vi "App - analyze RUS V6.vi"() -> ()   [LabVIEW 2021] (continued)
"temperature str"="160.67400", "file path"=path "D:/Data/Ultrasound/LSCO/LSCO22__130814c/5_Cooling_2nd_try/September_2014/091614/160.67400K_500_2500_2.10000V_0.00000T_Sep16-2014__16-59-49_001_091614.bin", "last mod"=timestamp(3493745989 s since 1904-01-01), "file name str"="D:\\Data\\Ultrasound\\LSCO\\LSCO22__130814c\\5_Cooling_2nd_try\\September_2014\\091614\\160.67400K_500_2500_2.10000V_0.00000T_Sep16-2014__16-59-49_001_091614.bin", "mod time(min)"=58229099.81666667, "file format"=enum."binary", "power(V)"=2.1, "Magn Field(T) "=0.0}, {"temperature"=160.342, "temperature str"="160.34200", "file path"=path "D:/Data/Ultrasound/LSCO/LSCO22__130814c/5_Cooling_2nd_try/September_2014/091614/160.34200K_500_2500_2.10000V_0.00000T_Sep16-2014__17-01-09_001_091614.bin", "last mod"=timestamp(3493746069 s since 1904-01-01), "file name str"="D:\\Data\\Ultrasound\\LSCO\\LSCO22__130814c\\5_Cooling_2nd_try\\September_2014\\091614\\160.34200K_500_2500_2.10000V_0.00000T_Sep16-2014__17-01-09_001_091614.bin", "mod time(min)"=58229101.15, "file format"=enum."binary", "power(V)"=2.1, "Magn Field(T) "=0.0}, {"temperature"=159.993, "temperature str"="159.99300", "file path"=path "D:/Data/Ultrasound/LSCO/LSCO22__130814c/5_Cooling_2nd_try/September_2014/091614/159.99300K_500_2500_2.10000V_0.00000T_Sep16-2014__17-02-28_001_091614.bin", "last mod"=timestamp(3493746148 s since 1904-01-01), "file name str"="D:\\Data\\Ultrasound\\LSCO\\LSCO22__130814c\\5_Cooling_2nd_try\\September_2014\\091614\\159.99300K_500_2500_2.10000V_0.00000T_Sep16-2014__17-02-28_001_091614.bin", "mod time(min)"=58229102.46666667, "file format"=enum."binary", "power(V)"=2.1, "Magn Field(T) "=0.0}, {"temperature"=159.648, "temperature str"="159.64800", "file path"=path "D:/Data/Ultrasound/LSCO/LSCO22__130814c/5_Cooling_2nd_try/September_2014/091614/159.64800K_500_2500_2.10000V_0.00000T_Sep16-2014__17-03-48_001_091614.bin", "last mod"=timestamp(3493746228 s since 1904-01-01), "file name str"="D:\\Data\\Ultrasound\\LSCO\\LSCO22__130814c\\5_Cooling_2nd_try\\September_2014\\091614\\159.64800K_500_2500_2.10000V_0.00000T_Sep16-2014__17-03-48_001_091614.bin", "mod time(min)"=58229103.8, "file format"=enum."binary", "power(V)"=2.1, "Magn Field(T) "=0.0}, {"temperature"=159.311, "temperature str"="159.31100", "file path"=path "D:/Data/Ultrasound/LSCO/LSCO22__130814c/5_Cooling_2nd_try/September_2014/091614/159.31100K_500_2500_2.10000V_0.00000T_Sep16-2014__17-05-07_001_091614.bin", "last mod"=timestamp(3493746307 s since 1904-01-01), "file name str"="D:\\Data\\Ultrasound\\LSCO\\LSCO22__130814c\\5_Cooling_2nd_try\\September_2014\\091614\\159.31100K_500_2500_2.10000V_0.00000T_Sep16-2014__17-05-07_001_091614.bin", "mod time(min)"=58229105.11666667, "file format"=enum."binary", "power(V)"=2.1, "Magn Field(T) "=0.0}, {"temperature"=158.97, "temperature str"="158.97000", "file path"=path "D:/Data/Ultrasound/LSCO/LSCO22__130814c/5_Cooling_2nd_try/September_2014/091614/158.97000K_500_2500_2.10000V_0.00000T_Sep16-2014__17-06-26_001_091614.bin", "last mod"=timestamp(3493746386 s since 1904-01-01), "file name str"="D:\\Data\\Ultrasound\\LSCO\\LSCO22__130814c\\5_Cooling_2nd_try\\September_2014\\091614\\158.97000K_500_2500_2.10000V_0.00000T_Sep16-2014__17-06-26_001_091614.bin", "mod time(min)"=58229106.43333333, "file format"=enum."binary", "power(V)"=2.1, "Magn Field(T) "=0.0}, {"temperature"=158.635, "temperature str"="158.63500", "file path"=path "D:/Data/Ultrasound/LSCO/LSCO22__130814c/5_Cooling_2nd_try/September_2014/091614/158.63500K_500_2500_2.10000V_0.00000T_Sep16-2014__17-07-46_001_091614.bin", "last mod"=timestamp(3493746466 s since 1904-01-01), "file name str"="D:\\Data\\Ultrasound\\LSCO\\LSCO22__130814c\\5_Cooling_2nd_try\\September_2014\\091614\\158.63500K_500_2500_2.10000V_0.00000T_Sep16-2014__17-07-46_001_091614.bin", "mod time(min)"=58229107.766666666, "file format"=enum."binary", "power(V)"=2.1, "Magn Field(T) "=0.0}, {"temperature"=158.293, "temperature str"="158.29300", "file path"=path "D:/Data/Ultrasound/LSCO/LSCO22__130814c/5_Cooling_2nd_try/September_2014/091614/158.29300K_500_2500_2.10000V_0.00000T_Sep16-2014__17-09-05_001_091614.bin", "last mod"=timestamp(3493746545 s since 1904-01-01), "file name str"="D:\\Data\\Ultrasound\\LSCO\\LSCO22__130814c\\5_Cooling_2nd_try\\September_2014\\091614\\158.29300K_500_2500_2.10000V_0.00000T_Sep16-2014__17-09-05_001_091614.bin", "mod time(min)"=58229109.083333336, "file format"=enum."binary", "power(V)"=2.1, "Magn Field(T) "=0.0}, {"temperature"=157.95, "temperature str"="157.95000", "file path"=path "D:/Data/Ultrasound/LSCO/LSCO22__130814c/5_Cooling_2nd_try/September_2014/091614/157.95000K_500_2500_2.10000V_0.00000T_Sep16-2014__17-10-24_001_091614.bin", "last mod"=timestamp(3493746624 s since 1904-01-01), "file name str"="D:\\Data\\Ultrasound\\LSCO\\LSCO22__130814c\\5_Cooling_2nd_try\\September_2014\\091614\\157.95000K_500_2500_2.10000V_0.00000T_Sep16-2014__17-10-24_001_091614.bin", "mod time(min)"=58229110.4, "file format"=enum."binary", "power(V)"=2.1, "Magn Field(T) "=0.0}, {"temperature"=157.609, "temperature str"="157.60900", "file path"=path "D:/Data/Ultrasound/LSCO/LSCO22__130814c/5_Cooling_2nd_try/September_2014/091614/157.60900K_500_2500_2.10000V_0.00000T_Sep16-2014__17-11-44_001_091614.bin", "last mod"=timestamp(3493746704 s since 1904-01-01), "file name str"="D:\\Data\\Ultrasound\\LSCO\\LSCO22__130814c\\5_Cooling_2nd_try\\September_2014\\091614\\157.60900K_500_2500_2.10000V_0.00000T_Sep16-2014__17-11-44_001_091614.bin", "mod time(min)"=58229111.733333334, "file format"=enum."binary", "power(V)"=2.1, "Magn Field(T) "=0.0}, {"temperature"=157.261, "temperature str"="157.26100", "file path"=path "D:/Data/Ultrasound/LSCO/LSCO22__130814c/5_Cooling_2nd_try/September_2014/091614/157.26100K_500_2500_2.10000V_0.00000T_Sep16-2014__17-13-03_001_091614.bin", "last mod"=timestamp(3493746783 s since 1904-01-01), "file name str"="D:\\Data\\Ultrasound\\LSCO\\LSCO22__130814c\\5_Cooling_2nd_try\\September_2014\\091614\\157.26100K_500_2500_2.10000V_0.00000T_Sep16-2014__17-13-03_001_091614.bin", "mod time(min)"=58229113.05, "file format"=enum."binary", "power(V)"=2.1, "Magn Field(T) "=0.0}, {"temperature"=156.94, "temperature str"="156.94000", "file path"=path "D:/Data/Ultrasound/LSCO/LSCO22__130814c/5_Cooling_2nd_try/September_2014/091614/156.94000K_500_2500_2.10000V_0.00000T_Sep16-2014__17-14-23_001_091614.bin", "last mod"=timestamp(3493746863 s since 1904-01-01), "file name str"="D:\\Data\\Ultrasound\\LSCO\\LSCO22__130814c\\5_Cooling_2nd_try\\September_2014\\091614\\156.94000K_500_2500_2.10000V_0.00000T_Sep16-2014__17-14-23_001_091614.bin", "mod time(min)"=58229114.38333333, "file format"=enum."binary", "power(V)"=2.1, "Magn Field(T) "=0.0}, {"temperature"=156.59, "temperature str"="156.59000", "file path"=path "D:/Data/Ultrasound/LSCO/LSCO22__130814c/5_Cooling_2nd_try/September_2014/091614/156.59000K_500_2500_2.10000V_0.00000T_Sep16-2014__17-15-42_001_091614.bin", "last mod"=timestamp(3493746942 s since 1904-01-01), "file name str"="D:\\Data\\Ultrasound\\LSCO\\LSCO22__130814c\\5_Cooling_2nd_try\\September_2014\\091614\\156.59000K_500_2500_2.10000V_0.00000T_Sep16-2014__17-15-42_001_091614.bin", "mod time(min)"=58229115.7, "file format"=enum."binary", "power(V)"=2.1, "Magn Field(T) "=0.0}, {"temperature"=156.243, "temperature str"="156.24300", "file path"=path "D:/Data/Ultrasound/LSCO/LSCO22__130814c/5_Cooling_2nd_try/September_2014/091614/156.24300K_500_2500_2.10000V_0.00000T_Sep16-2014__17-17-01_001_091614.bin", "last mod"=timestamp(3493747021 s since 1904-01-01), "file name str"="D:\\Data\\Ultrasound\\LSCO\\LSCO22__130814c\\5_Cooling_2nd_try\\September_2014\\091614\\156.24300K_500_2500_2.10000V_0.00000T_Sep16-2014__17-17-01_001_091614.bin", "mod time(min)"=58229117.016666666, "file format"=enum."binary", "power(V)"=2.1, "Magn Field(T) "=0.0}, {"temperature"=155.917, "temperature str"="155.91700", "file path"=path "D:/Data/Ultrasound/LSCO/LSCO22__130814c/5_Cooling_2nd_try/September_2014/091614/155.91700K_500_2500_2.10000V_0.00000T_Sep16-2014__17-18-21_001_091614.bin", "last mod"=timestamp(3493747101 s since 1904-01-01), "file name str"="D:\\Data\\Ultrasound\\LSCO\\LSCO22__130814c\\5_Cooling_2nd_try\\September_2014\\091614\\155.91700K_500_2500_2.10000V_0.00000T_Sep16-2014__17-18-21_001_091614.bin", "mod time(min)"=58229118.35, "file format"=enum."binary", "power(V)"=2.1, "Magn Field(T) "=0.0}, {"temperature"=155.569, "temperature str"="155.56900", "file path"=path "D:/Data/Ultrasound/LSCO/LSCO22__130814c/5_Cooling_2nd_try/September_2014/091614/155.56900K_500_2500_2.10000V_0.00000T_Sep16-2014__17-19-40_001_091614.bin", "last mod"=timestamp(3493747180 s since 1904-01-01), "file name str"="D:\\Data\\Ultrasound\\LSCO\\LSCO22__130814c\\5_Cooling_2nd_try\\September_2014\\091614\\155.56900K_500_2500_2.10000V_0.00000T_Sep16-2014__17-19-40_001_091614.bin", "mod time(min)"=58229119.666666664, "file format"=enum."binary", "power(V)"=2.1, "Magn Field(T) "=0.0}, {"temperature"=155.24, "temperature str"="155.24000", "file path"=path "D:/Data/Ultrasound/LSCO/LSCO22__130814c/5_Cooling_2nd_try/September_2014/091614/155.24000K_500_2500_2.10000V_0.00000T_Sep16-2014__17-20-59_001_091614.bin", "last mod"=timestamp(3493747259 s since 1904-01-01), "file name str"="D:\\Data\\Ultrasound\\LSCO\\LSCO22__130814c\\5_Cooling_2nd_try\\September_2014\\091614\\155.24000K_500_2500_2.10000V_0.00000T_Sep16-2014__17-20-59_001_091614.bin", "mod time(min)"=58229120.983333334, "file format"=enum."binary", "power(V)"=2.1, "Magn Field(T) "=0.0}, {"temperature"=154.892, "temperature str"="154.89200", "file path"=path "D:/Data/Ultrasound/LSCO/LSCO22__130814c/5_Cooling_2nd_try/September_2014/091614/154.89200K_500_2500_2.10000V_0.00000T_Sep16-2014__17-22-19_001_091614.bin", "last mod"=timestamp(3493747339 s since 1904-01-01), "file name str"="D:\\Data\\Ultrasound\\LSCO\\LSCO22__130814c\\5_Cooling_2nd_try\\September_2014\\091614\\154.89200K_500_2500_2.10000V_0.00000T_Sep16-2014__17-22-19_001_091614.bin", "mod time(min)"=58229122.31666667, "file format"=enum."binary", "power(V)"=2.1, "Magn Field(T) "=0.0}, {"temperature"=154.55, "temperature str"="154.55000", "file path"=path "D:/Data/Ultrasound/LSCO/LSCO22__130814c/5_Cooling_2nd_try/September_2014/091614/154.55000K_500_2500_2.10000V_0.00000T_Sep16-2014__17-23-38_001_091614.bin", "last mod"=timestamp(3493747418 s since 1904-01-01), "file name str"="D:\\Data\\Ultrasound\\LSCO\\LSCO22__130814c\\5_Cooling_2nd_try\\September_2014\\091614\\154.55000K_500_2500_2.10000V_0.00000T_Sep16-2014__17-23-38_001_091614.bin", "mod time(min)"=58229123.63333333, "file format"=enum."binary", "power(V)"=2.1, "Magn Field(T) "=0.0}, {"temperature"=154.223, "temperature str"="154.22300", "file path"=path "D:/Data/Ultrasound/LSCO/LSCO22__130814c/5_Cooling_2nd_try/September_2014/091614/154.22300K_500_2500_2.10000V_0.00000T_Sep16-2014__17-24-58_001_091614.bin", "last mod"=timestamp(3493747498 s since 1904-01-01), "file name str"="D:\\Data\\Ultrasound\\LSCO\\LSCO22__130814c\\5_Cooling_2nd_try\\September_2014\\091614\\154.22300K_500_2500_2.10000V_0.00000T_Sep16-2014__17-24-58_001_091614.bin", "mod time(min)"=58229124.96666667, "file format"=enum."binary", "power(V)"=2.1, "Magn Field(T) "=0.0}, {"temperature"=153.877, "temperature str"="153.87700", "file path"=path "D:/Data/Ultrasound/LSCO/LSCO22__130814c/5_Cooling_2nd_try/September_2014/091614/153.87700K_500_2500_2.10000V_0.00000T_Sep16-2014__17-26-17_001_091614.bin", "last mod"=timestamp(3493747577 s since 1904-01-01), "file name str"="D:\\Data\\Ultrasound\\LSCO\\LSCO22__130814c\\5_Cooling_2nd_try\\September_2014\\091614\\153.87700K_500_2500_2.10000V_0.00000T_Sep16-2014__17-26-17_001_091614.bin", "mod time(min)"=58229126.28333333, "file format"=enum."binary", "power(V)"=2.1, "Magn Field(T) "=0.0}, {"temperature"=153.533, "temperature str"="153.53300", "file path"=path "D:/Data/Ultrasound/LSCO/LSCO22__130814c/5_Cooling_2nd_try/September_2014/091614/153.53300K_500_2500_2.10000V_0.00000T_Sep16-2014__17-27-36_001_091614.bin", "last mod"=timestamp(3493747656 s since 1904-01-01), "file name str"="D:\\Data\\Ultrasound\\LSCO\\LSCO22__130814c\\5_Cooling_2nd_try\\September_2014\\091614\\153.53300K_500_2500_2.10000V_0.00000T_Sep16-2014__17-27-36_001_091614.bin", "mod time(min)"=58229127.6, "file format"=enum."binary", "power(V)"=2.1, "Magn Field(T) "=0.0}, {"temperature"=153.206, "temperature str"="153.20600", "file path"=path "D:/Data/Ultrasound/LSCO/LSCO22__130814c/5_Cooling_2nd_try/September_2014/091614/153.20600K_500_2500_2.10000V_0.00000T_Sep16-2014__17-28-56_001_091614.bin", "last mod"=timestamp(3493747736 s since 1904-01-01), "file name str"="D:\\Data\\Ultrasound\\LSCO\\LSCO22__130814c\\5_Cooling_2nd_try\\September_2014\\091614\\153.20600K_500_2500_2.10000V_0.00000T_Sep16-2014__17-28-56_001_091614.bin", "mod time(min)"=58229128.93333333, "file format"=enum."binary", "power(V)"=2.1, "Magn Field(T) "=0.0}, {"temperature"=152.863, "temperature str"="152.86300", "file path"=path "D:/Data/Ultrasound/LSCO/LSCO22__130814c/5_Cooling_2nd_try/September_2014/091614/152.86300K_500_2500_2.10000V_0.00000T_Sep16-2014__17-30-15_001_091614.bin", "last mod"=timestamp(3493747815 s since 1904-01-01), "file name str"="D:\\Data\\Ultrasound\\LSCO\\LSCO22__130814c\\5_Cooling_2nd_try\\September_2014\\091614\\152.86300K_500_2500_2.10000V_0.00000T_Sep16-2014__17-30-15_001_091614.bin", "mod time(min)"=58229130.25, "file format"=enum."binary", "power(V)"=2.1, "Magn Field(T) "=0.0}, {"temperature"=152.533, "temperature str"="152.53300", "file path"=path "D:/Data/Ultrasound/LSCO/LSCO22__130814c/5_Cooling_2nd_try/September_2014/091614/152.53300K_500_2500_2.10000V_0.00000T_Sep16-2014__17-31-35_001_091614.bin", "last mod"=timestamp(3493747895 s since 1904-01-01), "file name str"="D:\\Data\\Ultrasound\\LSCO\\LSCO22__130814c\\5_Cooling_2nd_try\\September_2014\\091614\\152.53300K_500_2500_2.10000V_0.00000T_Sep16-2014__17-31-35_001_091614.bin", "mod time(min)"=58229131.583333336, "file format"=enum."binary", "power(V)"=2.1, "Magn Field(T) "=0.0}, {"temperature"=152.199, "temperature str"="152.19900", "file path"=path "D:/Data/Ultrasound/LSCO/LSCO22__130814c/5_Cooling_2nd_try/September_2014/091614/152.19900K_500_2500_2.10000V_0.00000T_Sep16-2014__17-32-54_001_091614.bin", "last mod"=timestamp(3493747974 s since 1904-01-01), "file name str"="D:\\Data\\Ultrasound\\LSCO\\LSCO22__130814c\\5_Cooling_2nd_try\\September_2014\\091614\\152.19900K_500_2500_2.10000V_0.00000T_Sep16-2014__17-32-54_001_091614.bin", "mod time(min)"=58229132.9, "file format"=enum."binary", "power(V)"=2.1, "Magn Field(T) "=0.0}, {"temperature"=151.853, "temperature str"="151.85300", "file path"=path "D:/Data/Ultrasound/LSCO/LSCO22__130814c/5_Cooling_2nd_try/September_2014/091614/151.85300K_500_2500_2.10000V_0.00000T_Sep16-2014__17-34-13_001_091614.bin", "last mod"=timestamp(3493748053 s since 1904-01-01), "file name str"="D:\\Data\\Ultrasound\\LSCO\\LSCO22__130814c\\5_Cooling_2nd_try\\September_2014\\091614\\151.85300K_500_2500_2.10000V_0.00000T_Sep16-2014__17-34-13_001_091614.bin", "mod time(min)"=58229134.21666667, "file format"=enum."binary", "power(V)"=2.1, "Magn Field(T) "=0.0}, {"temperature"=151.527, "temperature str"="151.52700", "file path"=path "D:/Data/Ultrasound/LSCO/LSCO22__130814c/5_Cooling_2nd_try/September_2014/091614/151.52700K_500_2500_2.10000V_0.00000T_Sep16-2014__17-35-33_001_091614.bin", "last mod"=timestamp(3493748133 s since 1904-01-01), "file name str"="D:\\Data\\Ultrasound\\LSCO\\LSCO22__130814c\\5_Cooling_2nd_try\\September_2014\\091614\\151.52700K_500_2500_2.10000V_0.00000T_Sep16-2014__17-35-33_001_091614.bin", "mod time(min)"=58229135.55, "file format"=enum."binary", "power(V)"=2.1, "Magn Field(T) "=0.0}, {"temperature"=151.178, "temperature str"="151.17800", "file path"=path "D:/Data/Ultrasound/LSCO/LSCO22__130814c/5_Cooling_2nd_try/September_2014/091614/151.17800K_500_2500_2.10000V_0.00000T_Sep16-2014__17-36-52_001_091614.bin", "last mod"=timestamp(3493748212 s since 1904-01-01), "file name str"="D:\\Data\\Ultrasound\\LSCO\\LSCO22__130814c\\5_Cooling_2nd_try\\September_2014\\091614\\151.17800K_500_2500_2.10000V_0.00000T_Sep16-2014__17-36-52_001_091614.bin", "mod time(min)"=58229136.86666667, "file format"=enum."binary", "power(V)"=2.1, "Magn Field(T) "=0.0}, {"temperature"=150.857, "temperature str"="150.85700", "file path"=path "D:/Data/Ultrasound/LSCO/LSCO22__130814c/5_Cooling_2nd_try/September_2014/091614/150.85700K_500_2500_2.10000V_0.00000T_Sep16-2014__17-38-11_001_091614.bin", "last mod"=timestamp(3493748291 s since 1904-01-01), "file name str"="D:\\Data\\Ultrasound\\LSCO\\LSCO22__130814c\\5_Cooling_2nd_try\\September_2014\\091614\\150.85700K_500_2500_2.10000V_0.00000T_Sep16-2014__17-38-11_001_091614.bin", "mod time(min)"=58229138.18333333, "file format"=enum."binary", "power(V)"=2.1, "Magn Field(T) "=0.0}, {"temperature"=150.523, "temperature str"="150.52300", "file path"=path "D:/Data/Ultrasound/LSCO/LSCO22__130814c/5_Cooling_2nd_try/September_2014/091614/150.52300K_500_2500_2.10000V_0.00000T_Sep16-2014__17-39-31_001_091614.bin", "last mod"=timestamp(3493748371 s since 1904-01-01), "file name str"="D:\\Data\\Ultrasound\\LSCO\\LSCO22__130814c\\5_Cooling_2nd_try\\September_2014\\091614\\150.52300K_500_2500_2.10000V_0.00000T_Sep16-2014__17-39-31_001_091614.bin", "mod time(min)"=58229139.516666666, "file format"=enum."binary", "power(V)"=2.1, "Magn Field(T) "=0.0}, {"temperature"=150.18, "temperature str"="150.18000", "file path"=path "D:/Data/Ultrasound/LSCO/LSCO22__130814c/5_Cooling_2nd_try/September_2014/091614/150.18000K_500_2500_2.10000V_0.00000T_Sep16-2014__17-40-50_001_091614.bin", "last mod"=timestamp(3493748450 s since 1904-01-01), "file name str"="D:\\Data\\Ultrasound\\LSCO\\LSCO22__130814c\\5_Cooling_2nd_try\\September_2014\\091614\\150.18000K_500_2500_2.10000V_0.00000T_Sep16-2014__17-40-50_001_091614.bin", "mod time(min)"=58229140.833333336, "file format"=enum."binary", "power(V)"=2.1, "Magn Field(T) "=0.0}, {"temperature"=149.856, "temperature str"="149.85600", "file path"=path "D:/Data/Ultrasound/LSCO/LSCO22__130814c/5_Cooling_2nd_try/September_2014/091614/149.85600K_500_2500_2.10000V_0.00000T_Sep16-2014__17-42-10_001_091614.bin", "last mod"=timestamp(3493748530 s since 1904-01-01), "file name str"="D:\\Data\\Ultrasound\\LSCO\\LSCO22__130814c\\5_Cooling_2nd_try\\September_2014\\091614\\149.85600K_500_2500_2.10000V_0.00000T_Sep16-2014__17-42-10_001_091614.bin", "mod time(min)"=58229142.166666664, "file format"=enum."binary", "power(V)"=2.1, "Magn Field(T) "=0.0}, {"temperature"=149.518, "temperature str"="149.51800", "file path"=path "D:/Data/Ultrasound/LSCO/LSCO22__130814c/5_Cooling_2nd_try/September_2014/091614/149.51800K_500_2500_2.10000V_0.00000T_Sep16-2014__17-43-29_001_091614.bin", "last mod"=timestamp(3493748609 s since 1904-01-01), "file name str"="D:\\Data\\Ultrasound\\LSCO\\LSCO22__130814c\\5_Cooling_2nd_try\\September_2014\\091614\\149.51800K_500_2500_2.10000V_0.00000T_Sep16-2014__17-43-29_001_091614.bin", "mod time(min)"=58229143.483333334, "file format"=enum."binary", "power(V)"=2.1, "Magn Field(T) "=0.0}, {"temperature"=149.197, "temperature str"="149.19700", "file path"=path "D:/Data/Ultrasound/LSCO/LSCO22__130814c/5_Cooling_2nd_try/September_2014/091614/149.19700K_500_2500_2.10000V_0.00000T_Sep16-2014__17-44-48_001_091614.bin", "last mod"=timestamp(3493748688 s since 1904-01-01), "file name str"="D:\\Data\\Ultrasound\\LSCO\\LSCO22__130814c\\5_Cooling_2nd_try\\September_2014\\091614\\149.19700K_500_2500_2.10000V_0.00000T_Sep16-2014__17-44-48_001_091614.bin", "mod time(min)"=58229144.8, "file format"=enum."binary", "power(V)"=2.1, "Magn Field(T) "=0.0}, {"temperature"=148.854, "temperature str"="148.85400", "file path"=path "D:/Data/Ultrasound/LSCO/LSCO22__130814c/5_Cooling_2nd_try/September_2014/091614/148.85400K_500_2500_2.10000V_0.00000T_Sep16-2014__17-46-08_001_091614.bin", "last mod"=timestamp(3493748768 s since 1904-01-01), "file name str"="D:\\Data\\Ultrasound\\LSCO\\LSCO22__130814c\\5_Cooling_2nd_try\\September_2014\\091614\\148.85400K_500_2500_2.10000V_0.00000T_Sep16-2014__17-46-08_001_091614.bin", "mod time(min)"=58229146.13333333, "file format"=enum."binary", "power(V)"=2.1, "Magn Field(T) "=0.0}, {"temperature"=148.52, "temperature str"="148.52000", "file path"=path "D:/Data/Ultrasound/LSCO/LSCO22__130814c/5_Cooling_2nd_try/September_2014/091614/148.52000K_500_2500_2.10000V_0.00000T_Sep16-2014__17-47-27_001_091614.bin", "last mod"=timestamp(3493748847 s since 1904-01-01), "file name str"="D:\\Data\\Ultrasound\\LSCO\\LSCO22__130814c\\5_Cooling_2nd_try\\September_2014\\091614\\148.52000K_500_2500_2.10000V_0.00000T_Sep16-2014__17-47-27_001_091614.bin", "mod time(min)"=58229147.45, "file format"=enum."binary", "power(V)"=2.1, "Magn Field(T) "=0.0}, {"temperature"=148.201, "temperature str"="148.20100", "file path"=path "D:/Data/Ultrasound/LSCO/LSCO22__130814c/5_Cooling_2nd_try/September_2014/091614/148.20100K_500_2500_2.10000V_0.00000T_Sep16-2014__17-48-46_001_091614.bin", "last mod"=timestamp(3493748926 s since 1904-01-01), "file name str"="D:\\Data\\Ultrasound\\LSCO\\LSCO22__130814c\\5_Cooling_2nd_try\\September_2014\\091614\\148.20100K_500_2500_2.10000V_0.00000T_Sep16-2014__17-48-46_001_091614.bin", "mod time(min)"=58229148.766666666, "file format"=enum."binary", "power(V)"=2.1, "Magn Field(T) "=0.0}, {"temperature"=147.858, "temperature str"="147.85800", "file path"=path "D:/Data/Ultrasound/LSCO/LSCO22__130814c/5_Cooling_2nd_try/September_2014/091614/147.85800K_500_2500_2.10000V_0.00000T_Sep16-2014__17-50-06_001_091614.bin", "last mod"=timestamp(3493749006 s since 1904-01-01), "file name str"="D:\\Data\\Ultrasound\\LSCO\\LSCO22__130814c\\5_Cooling_2nd_try\\September_2014\\091614\\147.85800K_500_2500_2.10000V_0.00000T_Sep16-2014__17-50-06_001_091614.bin", "mod time(min)"=58229150.1, "file format"=enum."binary", "power(V)"=2.1, "Magn Field(T) "=0.0}, {"temperature"=147.54, "temperature str"="147.54000", "file path"=path "D:/Data/Ultrasound/LSCO/LSCO22__130814c/5_Cooling_2nd_try/September_2014/091614/147.54000K_500_2500_2.10000V_0.00000T_Sep16-2014__17-51-25_001_091614.bin", "last mod"=timestamp(3493749085 s since 1904-01-01), "file name str"="D:\\Data\\Ultrasound\\LSCO\\LSCO22__130814c\\5_Cooling_2nd_try\\September_2014\\091614\\147.54000K_500_2500_2.10000V_0.00000T_Sep16-2014__17-51-25_001_091614.bin", "mod time(min)"=58229151.416666664, "file format"=enum."binary", "power(V)"=2.1, "Magn Field(T) "=0.0}, {"temperature"=147.208, "temperature str"="147.20800", "file path"=path "D:/Data/Ultrasound/LSCO/LSCO22__130814c/5_Cooling_2nd_try/September_2014/091614/147.20800K_500_2500_2.10000V_0.00000T_Sep16-2014__17-52-45_001_091614.bin", "last mod"=timestamp(3493749165 s since 1904-01-01), "file name str"="D:\\Data\\Ultrasound\\LSCO\\LSCO22__130814c\\5_Cooling_2nd_try\\September_2014\\091614\\147.20800K_500_2500_2.10000V_0.00000T_Sep16-2014__17-52-45_001_091614.bin", "mod time(min)"=58229152.75, "file format"=enum."binary", "power(V)"=2.1, "Magn Field(T) "=0.0}, {"temperature"=146.868, "temperature str"="146.86800", "file path"=path "D:/Data/Ultrasound/LSCO/LSCO22__130814c/5_Cooling_2nd_try/September_2014/091614/146.86800K_500_2500_2.10000V_0.00000T_Sep16-2014__17-54-04_001_091614.bin", "last mod"=timestamp(3493749244 s since 1904-01-01), "file name str"="D:\\Data\\Ultrasound\\LSCO\\LSCO22__130814c\\5_Cooling_2nd_try\\September_2014\\091614\\146.86800K_500_2500_2.10000V_0.00000T_Sep16-2014__17-54-04_001_091614.bin", "mod time(min)"=58229154.06666667, "file format"=enum."binary", "power(V)"=2.1, "Magn Field(T) "=0.0}, {"temperature"=146.551, "temperature str"="146.55100", "file path"=path "D:/Data/Ultrasound/LSCO/LSCO22__130814c/5_Cooling_2nd_try/September_2014/091614/146.55100K_500_2500_2.10000V_0.00000T_Sep16-2014__17-55-23_001_091614.bin", "last mod"=timestamp(3493749323 s since 1904-01-01), "file name str"="D:\\Data\\Ultrasound\\LSCO\\LSCO22__130814c\\5_Cooling_2nd_try\\September_2014\\091614\\146.55100K_500_2500_2.10000V_0.00000T_Sep16-2014__17-55-23_001_091614.bin", "mod time(min)"=58229155.38333333, "file format"=enum."binary", "power(V)"=2.1, "Magn Field(T) "=0.0}, {"temperature"=146.222, "temperature str"="146.22200", "file path"=path "D:/Data/Ultrasound/LSCO/LSCO22__130814c/5_Cooling_2nd_try/September_2014/091614/146.22200K_500_2500_2.10000V_0.00000T_Sep16-2014__17-56-43_001_091614.bin", "last mod"=timestamp(3493749403 s since 1904-01-01), "file name str"="D:\\Data\\Ultrasound\\LSCO\\LSCO22__130814c\\5_Cooling_2nd_try\\September_2014\\091614\\146.22200K_500_2500_2.10000V_0.00000T_Sep16-2014__17-56-43_001_091614.bin", "mod time(min)"=58229156.71666667, "file format"=enum."binary", "power(V)"=2.1, "Magn Field(T) "=0.0}, {"temperature"=145.898, "temperature str"="145.89800", "file path"=path "D:/Data/Ultrasound/LSCO/LSCO22__130814c/5_Cooling_2nd_try/September_2014/091614/145.89800K_500_2500_2.10000V_0.00000T_Sep16-2014__17-58-02_001_091614.bin", "last mod"=timestamp(3493749482 s since 1904-01-01), "file name str"="D:\\Data\\Ultrasound\\LSCO\\LSCO22__130814c\\5_Cooling_2nd_try\\September_2014\\091614\\145.89800K_500_2500_2.10000V_0.00000T_Sep16-2014__17-58-02_001_091614.bin", "mod time(min)"=58229158.03333333, "file format"=enum."binary", "power(V)"=2.1, "Magn Field(T) "=0.0}, {"temperature"=145.567, "temperature str"="145.56700", "file path"=path "D:/Data/Ultrasound/LSCO/LSCO22__130814c/5_Cooling_2nd_try/September_2014/091614/145.56700K_500_2500_2.10000V_0.00000T_Sep16-2014__17-59-21_001_091614.bin", "last mod"=timestamp(3493749561 s since 1904-01-01), "file name str"="D:\\Data\\Ultrasound\\LSCO\\LSCO22__130814c\\5_Cooling_2nd_try\\September_2014\\091614\\145.56700K_500_2500_2.10000V_0.00000T_Sep16-2014__17-59-21_001_091614.bin", "mod time(min)"=58229159.35, "file format"=enum."binary", "power(V)"=2.1, "Magn Field(T) "=0.0}, {"temperature"=145.231, "temperature str"="145.23100", "file path"=path "D:/Data/Ultrasound/LSCO/LSCO22__130814c/5_Cooling_2nd_try/September_2014/091614/145.23100K_500_2500_2.10000V_0.00000T_Sep16-2014__18-00-41_001_091614.bin", "last mod"=timestamp(3493749641 s since 1904-01-01), "file name str"="D:\\Data\\Ultrasound\\LSCO\\LSCO22__130814c\\5_Cooling_2nd_try\\September_2014\\091614\\145.23100K_500_2500_2.10000V_0.00000T_Sep16-2014__18-00-41_001_091614.bin", "mod time(min)"=58229160.68333333, "file format"=enum."binary", "power(V)"=2.1, "Magn Field(T) "=0.0}, {"temperature"=144.914, "temperature str"="144.91400", "file path"=path "D:/Data/Ultrasound/LSCO/LSCO22__130814c/5_Cooling_2nd_try/September_2014/091614/144.91400K_500_2500_2.10000V_0.00000T_Sep16-2014__18-02-00_001_091614.bin", "last mod"=timestamp(3493749720 s since 1904-01-01), "file name str"="D:\\Data\\Ultrasound\\LSCO\\LSCO22__130814c\\5_Cooling_2nd_try\\September_2014\\091614\\144.91400K_500_2500_2.10000V_0.00000T_Sep16-2014__18-02-00_001_091614.bin", "mod time(min)"=58229162.0, "file format"=enum."binary", "power(V)"=2.1, "Magn Field(T) "=0.0}, {"temperature"=144.597, "temperature str"="144.59700", "file path"=path "D:/Data/Ultrasound/LSCO/LSCO22__130814c/5_Cooling_2nd_try/September_2014/091614/144.59700K_500_2500_2.10000V_0.00000T_Sep16-2014__18-03-20_001_091614.bin", "last mod"=timestamp(3493749800 s since 1904-01-01), "file name str"="D:\\Data\\Ultrasound\\LSCO\\LSCO22__130814c\\5_Cooling_2nd_try\\September_2014\\091614\\144.59700K_500_2500_2.10000V_0.00000T_Sep16-2014__18-03-20_001_091614.bin", "mod time(min)"=58229163.333333336, "file format"=enum."binary", "power(V)"=2.1, "Magn Field(T) "=0.0}, {"temperature"=144.27, "temperature str"="144.27000", "file path"=path "D:/Data/Ultrasound/LSCO/LSCO22__130814c/5_Cooling_2nd_try/September_2014/091614/144.27000K_500_2500_2.10000V_0.00000T_Sep16-2014__18-04-39_001_091614.bin", "last mod"=timestamp(3493749879 s since 1904-01-01), "file name str"="D:\\Data\\Ultrasound\\LSCO\\LSCO22__130814c\\5_Cooling_2nd_try\\September_2014\\091614\\144.27000K_500_2500_2.10000V_0.00000T_Sep16-2014__18-04-39_001_091614.bin", "mod time(min)"=58229164.65, "file format"=enum."binary", "power(V)"=2.1, "Magn Field(T) "=0.0}, {"temperature"=143.94, "temperature str"="143.94000", "file path"=path "D:/Data/Ultrasound/LSCO/LSCO22__130814c/5_Cooling_2nd_try/September_2014/091614/143.94000K_500_2500_2.10000V_0.00000T_Sep16-2014__18-05-58_001_091614.bin", "last mod"=timestamp(3493749958 s since 1904-01-01), "file name str"="D:\\Data\\Ultrasound\\LSCO\\LSCO22__130814c\\5_Cooling_2nd_try\\September_2014\\091614\\143.94000K_500_2500_2.10000V_0.00000T_Sep16-2014__18-05-58_001_091614.bin", "mod time(min)"=58229165.96666667, "file format"=enum."binary", "power(V)"=2.1, "Magn Field(T) "=0.0}, {"temperature"=143.619, "temperature str"="143.61900", "file path"=path "D:/Data/Ultrasound/LSCO/LSCO22__130814c/5_Cooling_2nd_try/September_2014/091614/143.61900K_500_2500_2.10000V_0.00000T_Sep16-2014__18-07-18_001_091614.bin", "last mod"=timestamp(3493750038 s since 1904-01-01), "file name str"="D:\\Data\\Ultrasound\\LSCO\\LSCO22__130814c\\5_Cooling_2nd_try\\September_2014\\091614\\143.61900K_500_2500_2.10000V_0.00000T_Sep16-2014__18-07-18_001_091614.bin", "mod time(min)"=58229167.3, "file format"=enum."binary", "power(V)"=2.1, "Magn Field(T) "=0.0}, {"temperature"=143.299, "temperature str"="143.29900", "file path"=path "D:/Data/Ultrasound/LSCO/LSCO22__130814c/5_Cooling_2nd_try/September_2014/091614/143.29900K_500_2500_2.10000V_0.00000T_Sep16-2014__18-08-37_001_091614.bin", "last mod"=timestamp(3493750117 s since 1904-01-01), "file name str"="D:\\Data\\Ultrasound\\LSCO\\LSCO22__130814c\\5_Cooling_2nd_try\\September_2014\\091614\\143.29900K_500_2500_2.10000V_0.00000T_Sep16-2014__18-08-37_001_091614.bin", "mod time(min)"=58229168.61666667, "file format"=enum."binary", "power(V)"=2.1, "Magn Field(T) "=0.0}, {"temperature"=142.977, "temperature str"="142.97700", "file path"=path "D:/Data/Ultrasound/LSCO/LSCO22__130814c/5_Cooling_2nd_try/September_2014/091614/142.97700K_500_2500_2.10000V_0.00000T_Sep16-2014__18-09-57_001_091614.bin", "last mod"=timestamp(3493750197 s since 1904-01-01), "file name str"="D:\\Data\\Ultrasound\\LSCO\\LSCO22__130814c\\5_Cooling_2nd_try\\September_2014\\091614\\142.97700K_500_2500_2.10000V_0.00000T_Sep16-2014__18-09-57_001_091614.bin", "mod time(min)"=58229169.95, "file format"=enum."binary", "power(V)"=2.1, "Magn Field(T) "=0.0}, {"temperature"=142.653, "temperature str"="142.65300", "file path"=path "D:/Data/Ultrasound/LSCO/LSCO22__130814c/5_Cooling_2nd_try/September_2014/091614/142.65300K_500_2500_2.10000V_0.00000T_Sep16-2014__18-11-16_001_091614.bin", "last mod"=timestamp(3493750276 s since 1904-01-01), "file name str"="D:\\Data\\Ultrasound\\LSCO\\LSCO22__130814c\\5_Cooling_2nd_try\\September_2014\\091614\\142.65300K_500_2500_2.10000V_0.00000T_Sep16-2014__18-11-16_001_091614.bin", "mod time(min)"=58229171.266666666, "file format"=enum."binary", "power(V)"=2.1, "Magn Field(T) "=0.0}, {"temperature"=142.336, "temperature str"="142.33600", "file path"=path "D:/Data/Ultrasound/LSCO/LSCO22__130814c/5_Cooling_2nd_try/September_2014/091614/142.33600K_500_2500_2.10000V_0.00000T_Sep16-2014__18-12-35_001_091614.bin", "last mod"=timestamp(3493750355 s since 1904-01-01), "file name str"="D:\\Data\\Ultrasound\\LSCO\\LSCO22__130814c\\5_Cooling_2nd_try\\September_2014\\091614\\142.33600K_500_2500_2.10000V_0.00000T_Sep16-2014__18-12-35_001_091614.bin", "mod time(min)"=58229172.583333336, "file format"=enum."binary", "power(V)"=2.1, "Magn Field(T) "=0.0}, {"temperature"=142.011, "temperature str"="142.01100", "file path"=path "D:/Data/Ultrasound/LSCO/LSCO22__130814c/5_Cooling_2nd_try/September_2014/091614/142.01100K_500_2500_2.10000V_0.00000T_Sep16-2014__18-13-55_001_091614.bin", "last mod"=timestamp(3493750435 s since 1904-01-01), "file name str"="D:\\Data\\Ultrasound\\LSCO\\LSCO22__130814c\\5_Cooling_2nd_try\\September_2014\\091614\\142.01100K_500_2500_2.10000V_0.00000T_Sep16-2014__18-13-55_001_091614.bin", "mod time(min)"=58229173.916666664, "file format"=enum."binary", "power(V)"=2.1, "Magn Field(T) "=0.0}, {"temperature"=141.704, "temperature str"="141.70400", "file path"=path "D:/Data/Ultrasound/LSCO/LSCO22__130814c/5_Cooling_2nd_try/September_2014/091614/141.70400K_500_2500_2.10000V_0.00000T_Sep16-2014__18-15-14_001_091614.bin", "last mod"=timestamp(3493750514 s since 1904-01-01), "file name str"="D:\\Data\\Ultrasound\\LSCO\\LSCO22__130814c\\5_Cooling_2nd_try\\September_2014\\091614\\141.70400K_500_2500_2.10000V_0.00000T_Sep16-2014__18-15-14_001_091614.bin", "mod time(min)"=58229175.233333334, "file format"=enum."binary", "power(V)"=2.1, "Magn Field(T) "=0.0}, {"temperature"=141.376, "temperature str"="141.37600", "file path"=path "D:/Data/Ultrasound/LSCO/LSCO22__130814c/5_Cooling_2nd_try/September_2014/091614/141.37600K_500_2500_2.10000V_0.00000T_Sep16-2014__18-16-33_001_091614.bin", "last mod"=timestamp(3493750593 s since 1904-01-01), "file name str"="D:\\Data\\Ultrasound\\LSCO\\LSCO22__130814c\\5_Cooling_2nd_try\\September_2014\\091614\\141.37600K_500_2500_2.10000V_0.00000T_Sep16-2014__18-16-33_001_091614.bin", "mod time(min)"=58229176.55, "file format"=enum."binary", "power(V)"=2.1, "Magn Field(T) "=0.0}, {"temperature"=141.051, "temperature str"="141.05100", "file path"=path "D:/Data/Ultrasound/LSCO/LSCO22__130814c/5_Cooling_2nd_try/September_2014/091614/141.05100K_500_2500_2.10000V_0.00000T_Sep16-2014__18-17-53_001_091614.bin", "last mod"=timestamp(3493750673 s since 1904-01-01), "file name str"="D:\\Data\\Ultrasound\\LSCO\\LSCO22__130814c\\5_Cooling_2nd_try\\September_2014\\091614\\141.05100K_500_2500_2.10000V_0.00000T_Sep16-2014__18-17-53_001_091614.bin", "mod time(min)"=58229177.88333333, "file format"=enum."binary", "power(V)"=2.1, "Magn Field(T) "=0.0}, {"temperature"=140.75, "temperature str"="140.75000", "file path"=path "D:/Data/Ultrasound/LSCO/LSCO22__130814c/5_Cooling_2nd_try/September_2014/091614/140.75000K_500_2500_2.10000V_0.00000T_Sep16-2014__18-19-12_001_091614.bin", "last mod"=timestamp(3493750752 s since 1904-01-01), "file name str"="D:\\Data\\Ultrasound\\LSCO\\LSCO22__130814c\\5_Cooling_2nd_try\\September_2014\\091614\\140.75000K_500_2500_2.10000V_0.00000T_Sep16-2014__18-19-12_001_091614.bin", "mod time(min)"=58229179.2, "file format"=enum."binary", "power(V)"=2.1, "Magn Field(T) "=0.0}, {"temperature"=140.423, "temperature str"="140.42300", "file path"=path "D:/Data/Ultrasound/LSCO/LSCO22__130814c/5_Cooling_2nd_try/September_2014/091614/140.42300K_500_2500_2.10000V_0.00000T_Sep16-2014__18-20-32_001_091614.bin", "last mod"=timestamp(3493750832 s since 1904-01-01), "file name str"="D:\\Data\\Ultrasound\\LSCO\\LSCO22__130814c\\5_Cooling_2nd_try\\September_2014\\091614\\140.42300K_500_2500_2.10000V_0.00000T_Sep16-2014__18-20-32_001_091614.bin", "mod time(min)"=58229180.53333333, "file format"=enum."binary", "power(V)"=2.1, "Magn Field(T) "=0.0}, {"temperature"=140.113, "temperature str"="140.11300", "file path"=path "D:/Data/Ultrasound/LSCO/LSCO22__130814c/5_Cooling_2nd_try/September_2014/091614/140.11300K_500_2500_2.10000V_0.00000T_Sep16-2014__18-21-51_001_091614.bin", "last mod"=timestamp(3493750911 s since 1904-01-01), "file name str"="D:\\Data\\Ultrasound\\LSCO\\LSCO22__130814c\\5_Cooling_2nd_try\\September_2014\\091614\\140.11300K_500_2500_2.10000V_0.00000T_Sep16-2014__18-21-51_001_091614.bin", "mod time(min)"=58229181.85, "file format"=enum."binary", "power(V)"=2.1, "Magn Field(T) "=0.0}, {"temperature"=139.803, "temperature str"="139.80300", "file path"=path "D:/Data/Ultrasound/LSCO/LSCO22__130814c/5_Cooling_2nd_try/September_2014/091614/139.80300K_500_2500_2.10000V_0.00000T_Sep16-2014__18-23-10_001_091614.bin", "last mod"=timestamp(3493750990 s since 1904-01-01), "file name str"="D:\\Data\\Ultrasound\\LSCO\\LSCO22__130814c\\5_Cooling_2nd_try\\September_2014\\091614\\139.80300K_500_2500_2.10000V_0.00000T_Sep16-2014__18-23-10_001_091614.bin", "mod time(min)"=58229183.166666664, "file format"=enum."binary", "power(V)"=2.1, "Magn Field(T) "=0.0}, {"temperature"=139.474, "temperature str"="139.47400", "file path"=path "D:/Data/Ultrasound/LSCO/LSCO22__130814c/5_Cooling_2nd_try/September_2014/091614/139.47400K_500_2500_2.10000V_0.00000T_Sep16-2014__18-24-30_001_091614.bin", "last mod"=timestamp(3493751070 s since 1904-01-01), "file name str"="D:\\Data\\Ultrasound\\LSCO\\LSCO22__130814c\\5_Cooling_2nd_try\\September_2014\\091614\\139.47400K_500_2500_2.10000V_0.00000T_Sep16-2014__18-24-30_001_091614.bin", "mod time(min)"=58229184.5, "file format"=enum."binary", "power(V)"=2.1, "Magn Field(T) "=0.0}, {"temperature"=139.164, "temperature str"="139.16400", "file path"=path "D:/Data/Ultrasound/LSCO/LSCO22__130814c/5_Cooling_2nd_try/September_2014/091614/139.16400K_500_2500_2.10000V_0.00000T_Sep16-2014__18-25-49_001_091614.bin", "last mod"=timestamp(3493751149 s since 1904-01-01), "file name str"="D:\\Data\\Ultrasound\\LSCO\\LSCO22__130814c\\5_Cooling_2nd_try\\September_2014\\091614\\139.16400K_500_2500_2.10000V_0.00000T_Sep16-2014__18-25-49_001_091614.bin", "mod time(min)"=58229185.81666667, "file format"=enum."binary", "power(V)"=2.1, "Magn Field(T) "=0.0}, {"temperature"=138.863, "temperature str"="138.86300", "file path"=path "D:/Data/Ultrasound/LSCO/LSCO22__130814c/5_Cooling_2nd_try/September_2014/091614/138.86300K_500_2500_2.10000V_0.00000T_Sep16-2014__18-27-09_001_091614.bin", "last mod"=timestamp(3493751229 s since 1904-01-01), "file name str"="D:\\Data\\Ultrasound\\LSCO\\LSCO22__130814c\\5_Cooling_2nd_try\\September_2014\\091614\\138.86300K_500_2500_2.10000V_0.00000T_Sep16-2014__18-27-09_001_091614.bin", "mod time(min)"=58229187.15, "file format"=enum."binary", "power(V)"=2.1, "Magn Field(T) "=0.0}, {"temperature"=138.548, "temperature str"="138.54800", "file path"=path "D:/Data/Ultrasound/LSCO/LSCO22__130814c/5_Cooling_2nd_try/September_2014/091614/138.54800K_500_2500_2.10000V_0.00000T_Sep16-2014__18-28-28_001_091614.bin", "last mod"=timestamp(3493751308 s since 1904-01-01), "file name str"="D:\\Data\\Ultrasound\\LSCO\\LSCO22__130814c\\5_Cooling_2nd_try\\September_2014\\091614\\138.54800K_500_2500_2.10000V_0.00000T_Sep16-2014__18-28-28_001_091614.bin", "mod time(min)"=58229188.46666667, "file format"=enum."binary", "power(V)"=2.1, "Magn Field(T) "=0.0}, {"temperature"=138.231, "temperature str"="138.23100", "file path"=path "D:/Data/Ultrasound/LSCO/LSCO22__130814c/5_Cooling_2nd_try/September_2014/091614/138.23100K_500_2500_2.10000V_0.00000T_Sep16-2014__18-29-47_001_091614.bin", "last mod"=timestamp(3493751387 s since 1904-01-01), "file name str"="D:\\Data\\Ultrasound\\LSCO\\LSCO22__130814c\\5_Cooling_2nd_try\\September_2014\\091614\\138.23100K_500_2500_2.10000V_0.00000T_Sep16-2014__18-29-47_001_091614.bin", "mod time(min)"=58229189.78333333, "file format"=enum."binary", "power(V)"=2.1, "Magn Field(T) "=0.0}, {"temperature"=137.923, "temperature str"="137.92300", "file path"=path "D:/Data/Ultrasound/LSCO/LSCO22__130814c/5_Cooling_2nd_try/September_2014/091614/137.92300K_500_2500_2.10000V_0.00000T_Sep16-2014__18-31-07_001_091614.bin", "last mod"=timestamp(3493751467 s since 1904-01-01), "file name str"="D:\\Data\\Ultrasound\\LSCO\\LSCO22__130814c\\5_Cooling_2nd_try\\September_2014\\091614\\137.92300K_500_2500_2.10000V_0.00000T_Sep16-2014__18-31-07_001_091614.bin", "mod time(min)"=58229191.11666667, "file format"=enum."binary", "power(V)"=2.1, "Magn Field(T) "=0.0}, {"temperature"=137.615, "temperature str"="137.61500", "file path"=path "D:/Data/Ultrasound/LSCO/LSCO22__130814c/5_Cooling_2nd_try/September_2014/091614/137.61500K_500_2500_2.10000V_0.00000T_Sep16-2014__18-32-26_001_091614.bin", "last mod"=timestamp(3493751546 s since 1904-01-01), "file name str"="D:\\Data\\Ultrasound\\LSCO\\LSCO22__130814c\\5_Cooling_2nd_try\\September_2014\\091614\\137.61500K_500_2500_2.10000V_0.00000T_Sep16-2014__18-32-26_001_091614.bin", "mod time(min)"=58229192.43333333, "file format"=enum."binary", "power(V)"=2.1, "Magn Field(T) "=0.0}, {"temperature"=137.3, "temperature str"="137.30000", "file 
